vi "Actor Core.vi"(8 "error in":errorcluster, 11 "GUARDAR_CSV in":refnum<class "GUARDAR_CSV.lvclass">) -> (0 "error out":errorcluster, 3 "Actor out":refnum<class "Actor.lvclass">)   [LabVIEW 2019, in "GUARDAR_CSV.lvlib" / "GUARDAR_CSV.lvclass"]
doc: "(<B>Filename</B>: Actor Framework.lvlib:Actor.lvclass:Actor Core.vi)\n\nReceives messages to the actor, reacts to them, and initiates any error handling that may shut the actor down.\n\nDescendant classes may override this VI to append parallel tasks for the actor to complete while it handles messages. Overrides use the Call Parent Method node."
uses:
  GUARDAR_CSV.lvclass
  <vilib>/ActorFramework/Actor/Actor.lvclass
  GUARDAR_CSV.lvclass/GUARDAR_CSV.ctl
panel:
  out "DATO":string
  out "Path":path
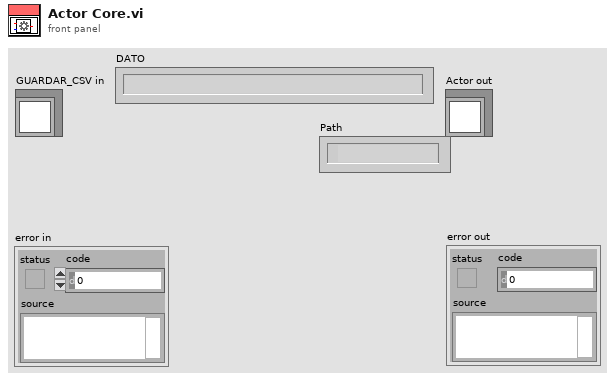
[diagram p1: front panel]
types:
  T1 = cluster{"Path":path, "PROVIENE DE?":enum16{"CONTADOR", "GENERADOR F"}, "DATO":string}
  T2 = cluster{"GUARDAR?":refnum<user-event>, "Path":refnum<user-event>, "PROVIENE DE?":refnum<user-event>, "EXIT":refnum<user-event>, "DATO":refnum<user-event>}
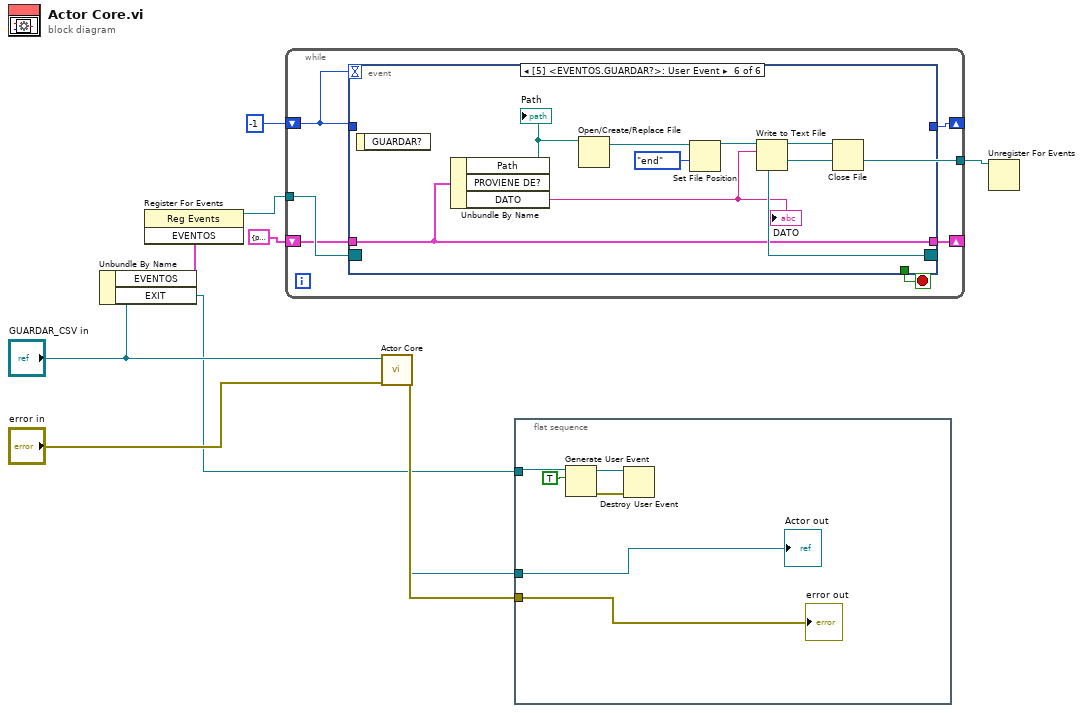
[diagram p0: block diagram]
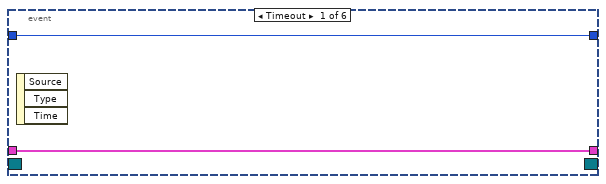
[diagram p2: hidden frame]
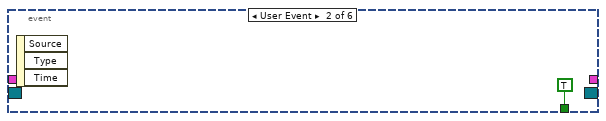
[diagram p3: hidden frame]
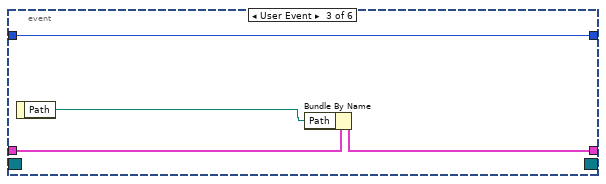
[diagram p4: hidden frame]
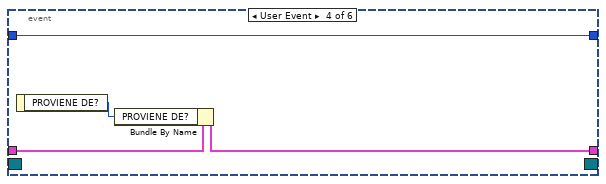
[diagram p5: hidden frame]
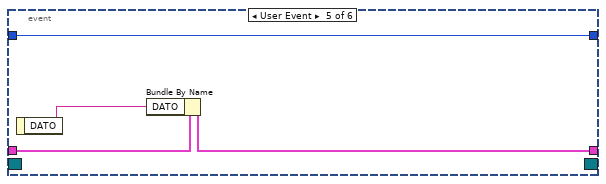
[diagram p6: hidden frame]
diagram:
  n1 = Unbundle By Name("GUARDAR_CSV in") -> ("EVENTOS"=w6:T2, "EXIT"=w4:refnum<user-event>)
  n2 = register-events(w6) -> (reference out=w5:refnum<event-registration>)  [unwired: 2 in, 1 out]
  n3 = while {
    tunnel: w5 -> [w17]
    tunnel: [w15] -> w3
    shift-right: [w14] -> _
    shift-left: -1 -> [w11]
    shift-right: [w12] -> _
    shift-left: T1 {"Path"=path "", "PROVIENE DE?"=enum."CONTADOR", "DATO"=""} -> [w13]
    stop <- w16 stop-if-true
    n4 = event shown="[5] <EVENTOS.GUARDAR?>: User Event" {
      selector: w17 -> [_ _ _ _ _ _]
      dyn-events: [_ _ _ _ _ _] -> w15
      timeout: w11 -> [_ _ _ _ _ _]
      tunnel: [_ TRUE _ _ _ _] -> w16
      tunnel: w11 -> [w19 _ w24 w27 w29 _]
      tunnel: [w19 _ w24 w27 w29 _] -> w14
      tunnel: w13 -> [w18 _ w23 w28 w32 w35]
      tunnel: [w18 _ w22 w26 w31 w35] -> w12
      event Timeout {
        n5 = event-data() -> ()  [unwired: 1 in, 3 out]
      }
      event User Event {
        n6 = event-data() -> ()  [unwired: 1 in, 3 out]
      }
      event User Event {
        n7 = event-data() -> ("Path"=w21:path)  [unwired: 1 in]
        n8 = Bundle By Name(cluster=w23, "Path"=w21) -> (w22:T1)
      }
      event User Event {
        n9 = event-data() -> ("PROVIENE DE?"=w25:enum16{"CONTADOR", "GENERADOR F"})  [unwired: 1 in]
        n10 = Bundle By Name(cluster=w28, "PROVIENE DE?"=w25) -> (w26:T1)
      }
      event User Event {
        n11 = event-data() -> ("DATO"=w30:string)  [unwired: 1 in]
        n12 = Bundle By Name(cluster=w32, "DATO"=w30) -> (w31:T1)
      }
      event User Event {
        n13 = event-data() -> ()  [unwired: 1 in, 1 out]
        n14 = Unbundle By Name(w35) -> ("Path"=w34:path, "DATO"=w33:string)  [unwired: 1 out]
        "Path" <- w34
        "DATO" <- w33
        n15 = Open/Create/Replace File(file path (use dialog)=w34) -> (refnum out=w39:refnum<file>)  [unwired: 5 in, 2 out]
        n16 = Set File Position(refnum=w39, from (0:start)=enum16{"start", "end", "current"}."end") -> (refnum out=w38:refnum<file>)  [unwired: 2 in, 1 out]
        n17 = Write to Text File(file (use dialog)=w38, text=w33) -> (refnum out=w37:refnum<file>)  [unwired: 2 in, 2 out]
        n18 = Close File(refnum=w37) -> ()  [unwired: 1 in, 2 out]
      }
    }
  }
  n19 = call-parent "Actor Core.vi"("error in"="error in", "Actor in"="GUARDAR_CSV in") -> ("error out"=w10:errorcluster, "Actor out"=w9:refnum<class "Actor.lvclass">)  [unwired: 8 in]
  n20 = flat-sequence {
    tunnel: w10 -> [w45]
    tunnel: w9 -> [w44]
    tunnel: w4 -> [w43]
    frame #0 {
      n21 = Generate User Event(user event=w43, event data cluster=TRUE ("event data")) -> (user event out=w40:refnum<user-event>, error out=w41:errorcluster)  [unwired: 2 in]
      n22 = Destroy User Event(user event=w40, error in=w41) -> ()  [unwired: 1 out]
      "error out" <- w45
      "Actor out" <- w44
    }
  }
  n23 = Unregister For Events(event registration refnum=w3) -> ()  [unwired: 1 in, 1 out]
